vi "CreateMissionWaypoints.vi"(5 "error in (no error)":errorcluster, 7 "WayPointCluster":T2 {"Drive Location"."North" format="%#_10f"; "Drive Location"."East" format="%#_8f"}, 8 "GoToWaypoint In":refnum<class "GoToWaypoint.lvclass">) -> (0 "error out":errorcluster, 3 "GoToWaypoint Out":refnum<class "GoToWaypoint.lvclass">)   [LabVIEW 2012, in "GoToWaypoint.lvclass"]
uses:
  GoToWaypoint.lvclass
  Sailbot2012_2013/Software/2-Think/2 Typedefs/UTM Location.ctl
  GoToWaypoint.lvclass/GoToWaypoint.ctl
  Sailbot2012_2013/Software/2-Think/2 Classes/Waypoint/Waypoint.lvclass
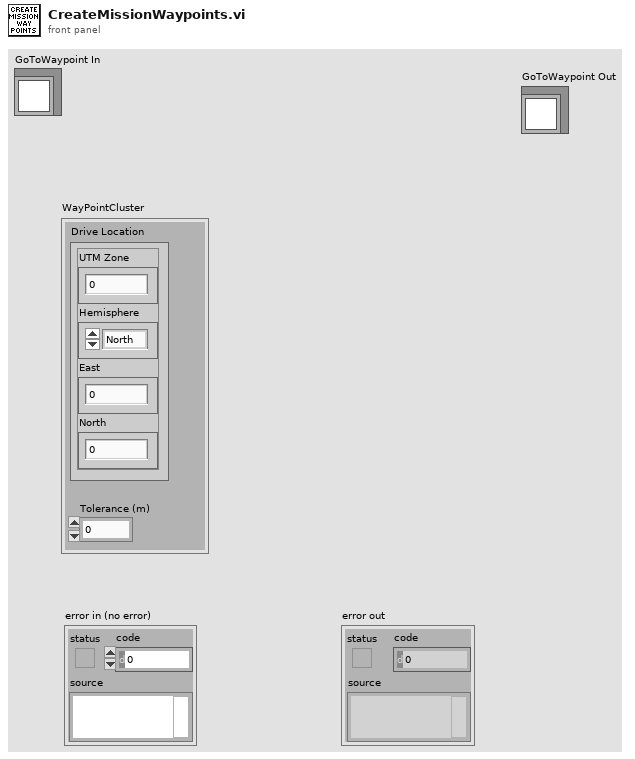
[diagram p1: front panel]
types:
  T1 = typedef "UTM Location.ctl" = cluster{"UTM Zone":dbl, "Hemisphere":enum16{"North", "South"}, "East":dbl, "North":dbl}
  T2 = cluster{"Drive Location":T1, "Tolerance (m)":dbl}
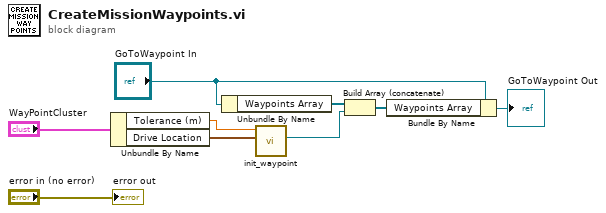
[diagram p0: block diagram]
diagram:
  n1 = Unbundle By Name("WayPointCluster") -> ("Tolerance (m)"=w5:dbl, "Drive Location"=w9:T1)
  n2 = Unbundle By Name("GoToWaypoint In") -> ("Waypoints Array"=w4:refnum<class "Waypoint.lvclass">[])
  n3 = call "init_waypoint.vi"("Coords"=w9, "Tolerance (m)"=w5) -> ("Waypoint Out"=w8:refnum<class "Waypoint.lvclass">)  [unwired: 9 in]
  n4 = Build Array (concatenate)(w4, w8) -> (w3:refnum<class "Waypoint.lvclass">[])
  n5 = Bundle By Name(cluster="GoToWaypoint In", "Waypoints Array"=w3) -> (→"GoToWaypoint Out":refnum<class "GoToWaypoint.lvclass">)
  "error out" <- "error in (no error)"
